vi "Resize.Resize Unstacked Plot Chart within Tab Ctrl.vi"(4 "Plot Cnt":i32=4, 5 "Pix from Bottom":i32, 6 "Min Size":cluster{"Width":i32, "Height":i32}={"Width"=250, "Height"=200}, 7 "Pix from Right":i32, 8 "error in":errorcluster, 9 "Aspect Ratio":cluster{"W/H":dbl, "Enable":bool}={"W/H"=1.0, "Enable"=FALSE} {"W/H" format="%.2g"}, 10 "Chart Ctrl":refnum<vi>, 11 "Tab Ctrl":refnum<vi>) -> (0 "error out":errorcluster, 2 "Chart Ctrl Out":refnum<vi>, 3 "Tab Ctrl Out":refnum<vi>)   [LabVIEW 2024, in "EQMF.lvlib" / "Controls.lvlib"]
uses:
  Controls.lvlib
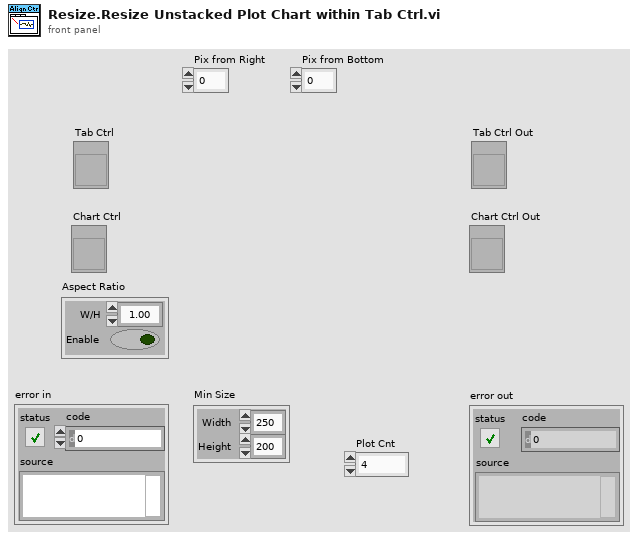
[diagram p1: front panel]
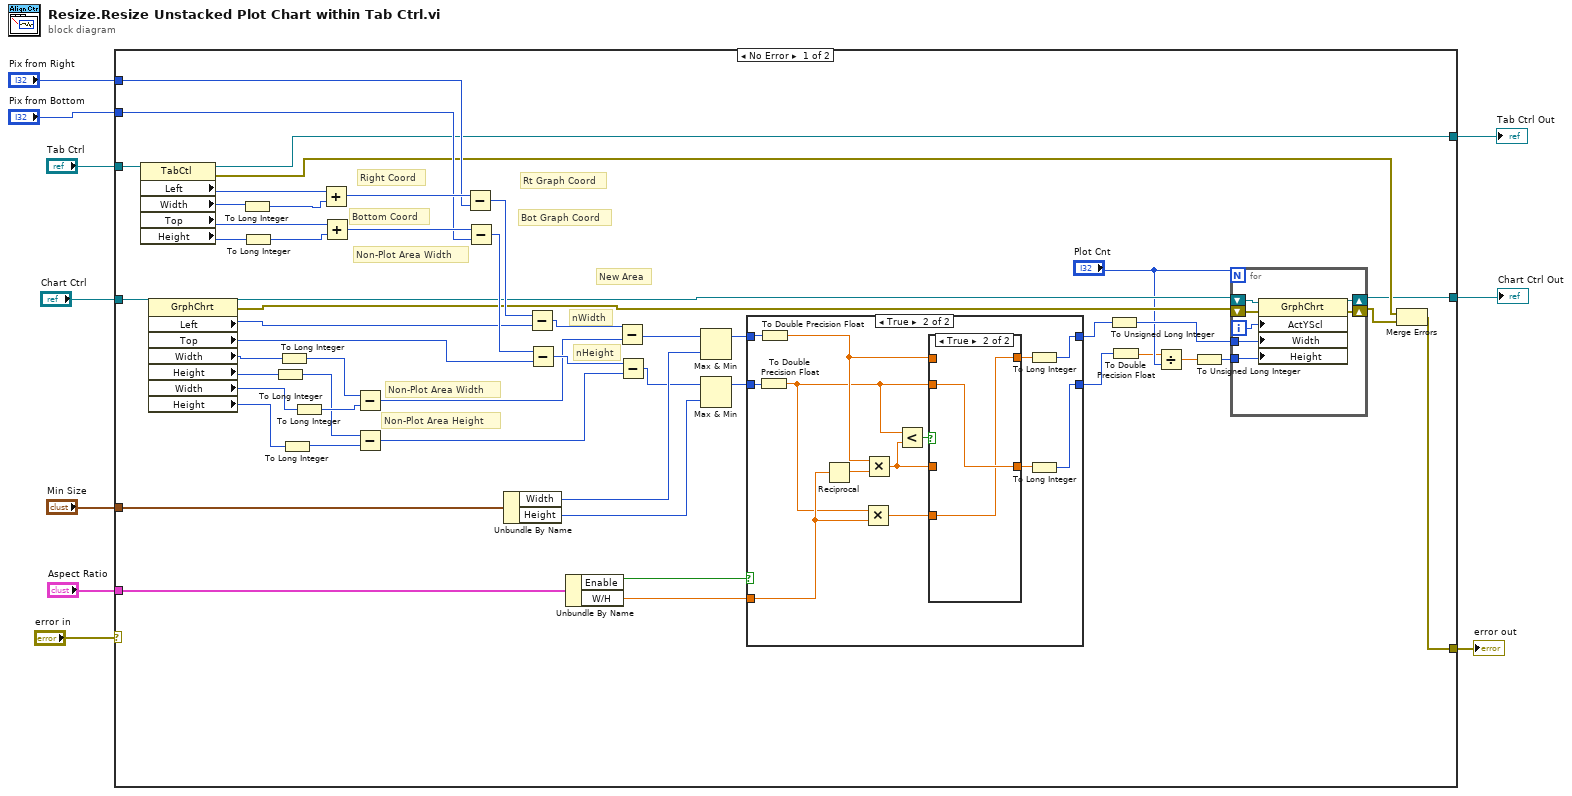
[diagram p0: block diagram]
diagram:
  n1 = case shown="No Error" "error in" {
    selector: "error in" -> [_ w89]
    tunnel: "Pix from Right" -> [w46 _]
    tunnel: "Pix from Bottom" -> [w45 _]
    tunnel: [w34 w89] -> w8
    tunnel: "Min Size" -> [w33 _]
    tunnel: "Aspect Ratio" -> [w26 _]
    tunnel: "Tab Ctrl" -> [w23 w91]
    tunnel: "Chart Ctrl" -> [w22 w90]
    tunnel: [w19 w91] -> w3
    tunnel: [w18 w90] -> w2
    frame No Error {
      # "nHeight"
      # "nWidth"
      # "New Area"
      # "Bot Graph Coord"
      # "Rt Graph Coord"
      # "Non-Plot Area Width"
      # "Bottom Coord"
      # "Right Coord"
      # "Non-Plot Area Height"
      # "Non-Plot Area Width"
      n2 = property on="Property Node" class="TabCtl"(reference=w23) -> (reference out=w19:refnum<vi>, error out=w21:errorcluster, "Left"=w50:i32, "Width"=w53:u32, "Top"=w51:i32, "Height"=w52:u32)  [unwired: 1 in]
      n3 = property on="Property Node" class="GrphChrt"(reference=w22) -> (reference out=w36:refnum<vi>, error out=w35:errorcluster, "Left"=w42:i32, "Top"=w41:i32, "Width"=w49:u32, "Height"=w62:u32, "Width"=w61:u32, "Height"=w60:u32)  [unwired: 1 in]
      n4 = To Long Integer(number=w53) -> (32bit integer=w54:i32)
      n5 = To Long Integer(number=w52) -> (32bit integer=w55:i32)
      n6 = To Long Integer(number=w62) -> (32bit integer=w57:i32)
      n7 = To Long Integer(number=w49) -> (32bit integer=w58:i32)
      n8 = To Long Integer(number=w60) -> (32bit integer=w56:i32)
      n9 = To Long Integer(number=w61) -> (32bit integer=w59:i32)
      n10 = Add(x=w50, y=w54) -> (x+y=w47:i32)
      n11 = Add(x=w51, y=w55) -> (x+y=w48:i32)
      n12 = Subtract(x=w58, y=w59) -> (x-y=w38:i32)
      n13 = Subtract(x=w57, y=w56) -> (x-y=w37:i32)
      n14 = Subtract(x=w47, y=w46) -> (x-y=w44:i32)
      n15 = Subtract(x=w48, y=w45) -> (x-y=w43:i32)
      n16 = Unbundle By Name(w33) -> ("Width"=w32:i32, "Height"=w31:i32)
      n17 = Subtract(x=w44, y=w42) -> (x-y=w40:i32)
      n18 = Subtract(x=w43, y=w41) -> (x-y=w39:i32)
      n19 = Unbundle By Name(w26) -> ("Enable"=w25:bool, "W/H"=w24:dbl)
      n20 = Subtract(x=w40, y=w38) -> (x-y=w29:i32)
      n21 = Subtract(x=w39, y=w37) -> (x-y=w30:i32)
      n22 = Max & Min(x=w29, y=w32) -> (max(x,y)=w28:i32)  [unwired: 1 out]
      n23 = Max & Min(x=w30, y=w31) -> (max(x,y)=w27:i32)  [unwired: 1 out]
      n24 = case shown="True" w25 {
        tunnel: w28 -> [w71 w84]
        tunnel: w27 -> [w70 w83]
        tunnel: [w71 w75] -> w17
        tunnel: [w70 w76] -> w13
        tunnel: w24 -> [_ w81]
        frame False {
        }
        frame True {
          n25 = To Double Precision Float(number=w83) -> (double precision float=w73:dbl)
          n26 = To Double Precision Float(number=w84) -> (double precision float=w80:dbl)
          n27 = Reciprocal(x=w81) -> (1/x=w82:dbl)
          n28 = Multiply(x=w73, y=w81) -> (x*y=w72:dbl)
          n29 = Multiply(x=w80, y=w82) -> (x*y=w79:dbl)
          n30 = Less?(x=w73, y=w79) -> (x < y?=w78:bool)
          n31 = case shown="True" w78 {
            tunnel: w80 -> [w86 _]
            tunnel: w79 -> [w85 _]
            tunnel: [w86 w87] -> w74
            tunnel: [w85 w88] -> w77
            tunnel: w73 -> [_ w88]
            tunnel: w72 -> [_ w87]
            frame False {
            }
            frame True {
            }
          }
          n32 = To Long Integer(number=w74) -> (32bit integer=w75:i32)
          n33 = To Long Integer(number=w77) -> (32bit integer=w76:i32)
        }
      }
      n34 = To Unsigned Long Integer(number=w17) -> (unsigned 32bit integer=w16:u32)
      n35 = To Double Precision Float(number=w13) -> (double precision float=w14:dbl)
      n36 = Divide(x=w14, y="Plot Cnt") -> (x/y=w11:dbl)
      n37 = To Unsigned Long Integer(number=w11) -> (unsigned 32bit integer=w12:u32)
      n38 = for {
        N: "Plot Cnt" -> [_]
        shift-right: [w66] -> w18
        shift-left: w36 -> [w69]
        shift-right: [w67] -> w20
        shift-left: w35 -> [w68]
        tunnel: w16 -> [w64]
        tunnel: w12 -> [w63]
        i -> [w65]
        n39 = property on="Property Node" class="GrphChrt"(reference=w69, error in=w68, "ActYScl"=w65, "Width"=w64, "Height"=w63) -> (reference out=w66:refnum<vi>, error out=w67:errorcluster)
      }
      n40 = Merge Errors(w21, w20) -> (w34:errorcluster)
    }
    frame Error {
    }
  }
  "error out" <- w8
  "Tab Ctrl Out" <- w3
  "Chart Ctrl Out" <- w2
